vi "Tosca-Evaluate Criterion.vi"(0 "Criterion":T1, 7 "Digital Inputs":T3[](array[typedef])) -> (8 "Criterion met?":bool)   [LabVIEW 2020]
uses:
  Tosca-Digital Input.ctl
  Tosca-Input Criterion.ctl
  epl-vi-lib/Utility VIs/Type Defs/Logic State.ctl
  Sub VIs/Tosca-Globals.vi
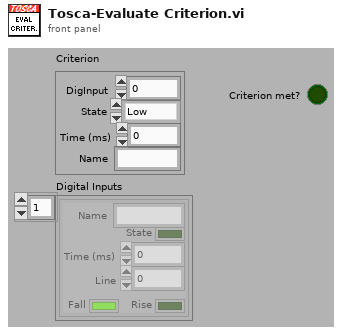
[diagram p1: front panel]
types:
  T1 = typedef "Tosca-Input Criterion.ctl" = cluster{"DigInput":i32, "State":T2, "Time (ms)":i32, "Name":string}
  T2 = typedef "Logic State.ctl" = enum16{"Low", "High", "Rising", "Falling"}
  T3 = typedef "Tosca-Digital Input.ctl" = cluster{"Name":string, "State":bool, "Time (ms)":dbl, "Line":i32, "Rise":bool, "Fall":bool}
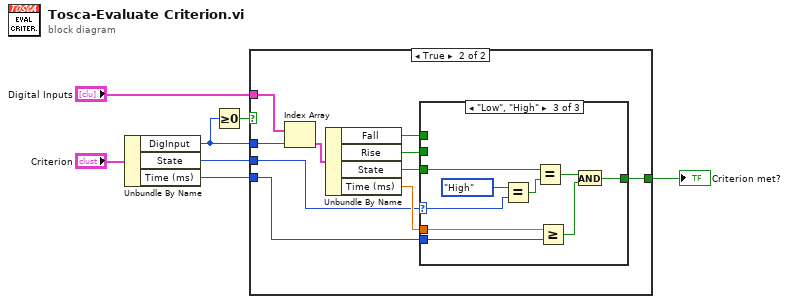
[diagram p0: block diagram]
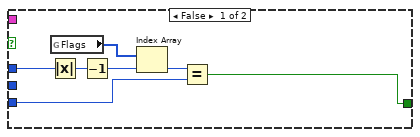
[diagram p2: hidden frame]
diagram:
  n1 = Unbundle By Name("Criterion") -> ("DigInput"=w3:i32, "State"=w1:T2, "Time (ms)"=w7:i32)
  n2 = Greater Or Equal To 0?(x=w3) -> (x >= 0?=w2:bool)
  n3 = case shown="True" w2 {
    tunnel: w7 -> [w9 w24]
    tunnel: "Digital Inputs" -> [_ w19]
    tunnel: w3 -> [w14 w17]
    tunnel: [w8 w21] -> w4
    tunnel: w1 -> [_ w18]
    frame False {
      n4 = Absolute Value(x=w14) -> (abs(x)=w13:i32)
      n5 = global read "Tosca-Globals.vi" "Flags"() -> (w11:i32[])
      n6 = Decrement(x=w13) -> (x-1=w12:i32)
      n7 = Index Array(array=w11, index=w12) -> (element=w10:i32)
      n8 = Equal?(x=w10, y=w9) -> (x = y?=w8:bool)
    }
    frame True {
      n9 = Index Array(array=w19, index=w17) -> (element=w22:T3)
      n10 = Unbundle By Name(w22) -> ("Fall"=w15:bool, "Rise"=w16:bool, "State"=w23:bool, "Time (ms)"=w20:dbl)
      n11 = case shown="\"Low\", \"High\"" w18 {
        selector: w18 -> [_ _ w28]
        tunnel: w24 -> [_ _ w33]
        tunnel: w23 -> [_ _ w32]
        tunnel: [w25 w26 w31] -> w21
        tunnel: w20 -> [_ _ w30]
        tunnel: w16 -> [w25 _ _]
        tunnel: w15 -> [_ w26 _]
        frame "Rising" {
        }
        frame "Falling" {
        }
        frame "Low", "High" {
          n12 = Equal?(x=Logic_State."High", y=w28) -> (x = y?=w29:bool)
          n13 = Equal?(x=w32, y=w29) -> (x = y?=w34:bool)
          n14 = Greater Or Equal?(x=w30, y=w33) -> (x >= y?=w35:bool)
          n15 = And(x=w34, y=w35) -> (x .and. y?=w31:bool)
        }
      }
    }
  }
  "Criterion met?" <- w4
